vi "NR Fetch ACP.vi"(0 "RFmx Handle In":refnum<k21>, 1 "Selector String":string, 11 "error in (no error)":errorcluster) -> (4 "RFmx Handle Out":refnum<k21>, 6 "ACP Results":T1, 15 "error out":errorcluster)   [LabVIEW 2016, in "RFmxNR.lvlib"]
uses:
  RFmxNR.lvlib
  Typedefs/NR ACP Results.ctl
  Typedefs/NR ACP Offset Results.ctl
  Typedefs/NR ACP Component Carrier Results.ctl
  <vilib>/RFmx/NR/mx/RFmxNR.llb/RFmxNR ACP Fetch Offset Measurement (Array).vi
  <vilib>/RFmx/NR/mx/RFmxNR.llb/RFmxNR ACP Fetch Component Carrier Measurement (Array).vi
  <resource>/objmgr/RFmxLTE.rc
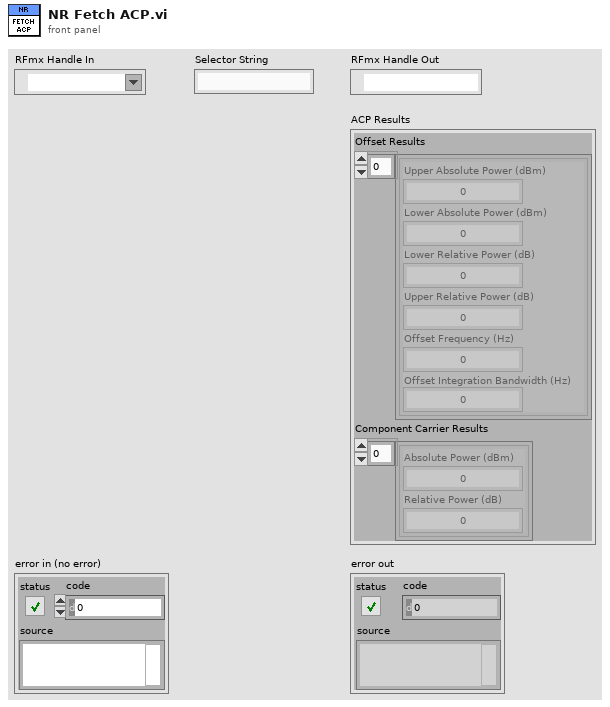
[diagram p1: front panel]
types:
  T1 = typedef "RFmxNR.lvlib/NR ACP Results.ctl" = cluster{"Offset Results":T2[], "Component Carrier Results":T3[]}
  T2 = typedef "RFmxNR.lvlib/NR ACP Offset Results.ctl" = cluster{"Upper Absolute Power (dBm)":dbl, "Lower Absolute Power (dBm)":dbl, "Lower Relative Power (dB)":dbl, "Upper Relative Power (dB)":dbl, "Offset Frequency (Hz)":dbl, "Offset Integration Bandwidth (Hz)":dbl}
  T3 = typedef "RFmxNR.lvlib/NR ACP Component Carrier Results.ctl" = cluster{"Absolute Power (dBm)":dbl, "Relative Power (dB)":dbl}
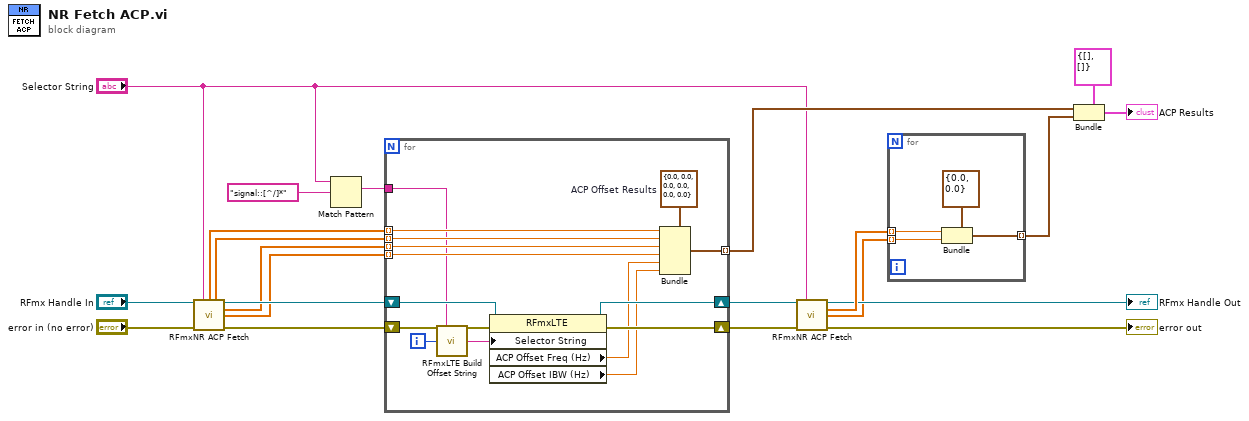
[diagram p0: block diagram]
diagram:
  n1 = call-poly <vilib>:"RFmxNR ACP Fetch.vi"("Instrument Handle In"="RFmx Handle In", "Selector String"="Selector String", "error in (no error)"="error in (no error)") -> ("Upper Absolute Power (dBm)"=w5:dbl[], "Lower Absolute Power (dBm)"=w17:dbl[], "Instrument Handle Out"=w19:refnum<k21>, "Lower Relative Power (dB)"=w16:dbl[], "Upper Relative Power (dB)"=w15:dbl[], "error out"=w18:errorcluster)  [unwired: 7 in]
  n2 = Match Pattern(string="Selector String", regular expression="signal::[^/]*") -> (match substring=w13:string)  [unwired: 1 in, 3 out]
  n3 = for {
    shift-right: [w34] -> w12
    shift-left: w19 -> [w28]
    shift-right: [w35] -> w11
    shift-left: w18 -> [w27]
    tunnel: [w30] -> w20 mode=indexing
    tunnel: w5 -> [w26] mode=indexing
    tunnel: w17 -> [w25] mode=indexing
    tunnel: w16 -> [w24] mode=indexing
    tunnel: w15 -> [w23] mode=indexing
    tunnel: w13 -> [w22]
    i -> [w36]
    w33 = T2 {"Upper Absolute Power (dBm)"=0.0, "Lower Absolute Power (dBm)"=0.0, "Lower Relative Power (dB)"=0.0, "Upper Relative Power (dB)"=0.0, "Offset Frequency (Hz)"=0.0, "Offset Integration Bandwidth (Hz)"=0.0}  # ACP Offset Results
    n4 = call <vilib>:"RFmxLTE Build Offset String.vi"("Selector String"=w22, "Offset Number"=w36) -> ("Selector String Out"=w29:string)  [unwired: 13 in]
    n5 = property class="RFmxLTE"(reference=w28, error in=w27, "Selector String"=w29) -> (reference out=w34:refnum<k21>, error out=w35:errorcluster, "ACP Offset Freq (Hz)"=w31:dbl, "ACP Offset IBW (Hz)"=w32:dbl)
    n6 = Bundle(cluster=w33, "Upper Absolute Power (dBm)"=w26, "Lower Absolute Power (dBm)"=w25, "Lower Relative Power (dB)"=w24, "Upper Relative Power (dB)"=w23, "Offset Frequency (Hz)"=w31, "Offset Integration Bandwidth (Hz)"=w32) -> (w30:T2)
  }
  n7 = call-poly <vilib>:"RFmxNR ACP Fetch.vi"("Instrument Handle In"=w12, "Selector String"="Selector String", "error in (no error)"=w11) -> ("Instrument Handle Out"=→"RFmx Handle Out":refnum<k21>, "Absolute Power (dBm)"=w10:dbl[], "Relative Power (dB)"=w3:dbl[], "error out"=→"error out":errorcluster)  [unwired: 9 in]
  n8 = for {
    tunnel: [w40] -> w21 mode=indexing
    tunnel: w10 -> [w39] mode=indexing
    tunnel: w3 -> [w38] mode=indexing
    n9 = Bundle(cluster=T3 {"Absolute Power (dBm)"=0.0, "Relative Power (dB)"=0.0} ("NR ACP Component Carrier Results"), "Absolute Power (dBm)"=w39, "Relative Power (dB)"=w38) -> (w40:T3)
  }
  n10 = Bundle(cluster=T1 {"Offset Results"=[], "Component Carrier Results"=[]} ("NR ACP Results"), "Offset Results"=w20, "Component Carrier Results"=w21) -> (→"ACP Results":T1)
